vi "Equal.vi"() -> ()   [LabVIEW 2017, in "Assertions.Tests.lvlib" / "Assert Greater Than or Equal To.lvlib"]
uses:
  Assert Greater Than or Equal To.lvlib
  2c547ce4-3ad5-460a-b43d-24432c77f328.vi
  src/Transparent Assertions/Constraints/Logical Or/Logical Or.lvclass
  C:/Users/pasca/Projects/Home/TransparentAssertions/src/Transparent Assertions/Constraints/Binary Operator/Binary Operator.lvclass
  src/Transparent Assertions/Constraints/IsEqual/IsEqual.lvclass
  C:/Users/pasca/Projects/Home/TransparentAssertions/src/Transparent Assertions/Constraints/Constraint/Constraint.lvclass
  src/Transparent Assertions/Constraints/Is Greater Than/Is Greater Than.lvclass
  src/Transparent Assertions/Constraints/IsEqual/Create.vi
  src/Transparent Assertions/Constraints/Is Greater Than/Create.vi
  src/Transparent Assertions/Constraints/Binary Operator/Create.vi
  src/Transparent Assertions/Assertions/Assertions.lvlib
panel:
  out "error out":errorcluster
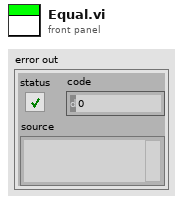
[diagram p1: front panel]
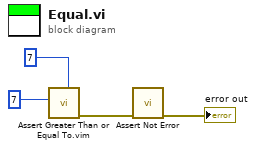
[diagram p0: block diagram]
diagram:
  n1 = call "Assert Greater Than or Equal To.vim"("Expected"=7, "Actual"=7) -> ("error out"=w2:errorcluster)  [unwired: 9 in]
  n2 = call "Assert Not Error.vi"("error in (no error)"=w2) -> ("error out"=→"error out":errorcluster)  [unwired: 10 in]
